vi "Draw Stats.vi"(10 "Stats":T1={"Transform And Project Duration"=0.0, "Raster Duration"=0.0, "Present Duration"=82.5692473, "Frame Rate"=111.70812900055276, "Visible Triangles"=0} {"Frame Rate" format="%.0p"; "Present Duration" format="%.0p"; "Raster Duration" format="%.0p"; "Transform And Project Duration" format="%.0p"}, 11 "Screen in":picture) -> (3 "Screen out":picture)   [LabVIEW 2022 SP3, in "Application.lvlib"]
uses:
  Application.lvlib
  Scene/Stats.ctl
  Libraries/Utility/Utility.lvlib
  Scene/Scene.lvclass
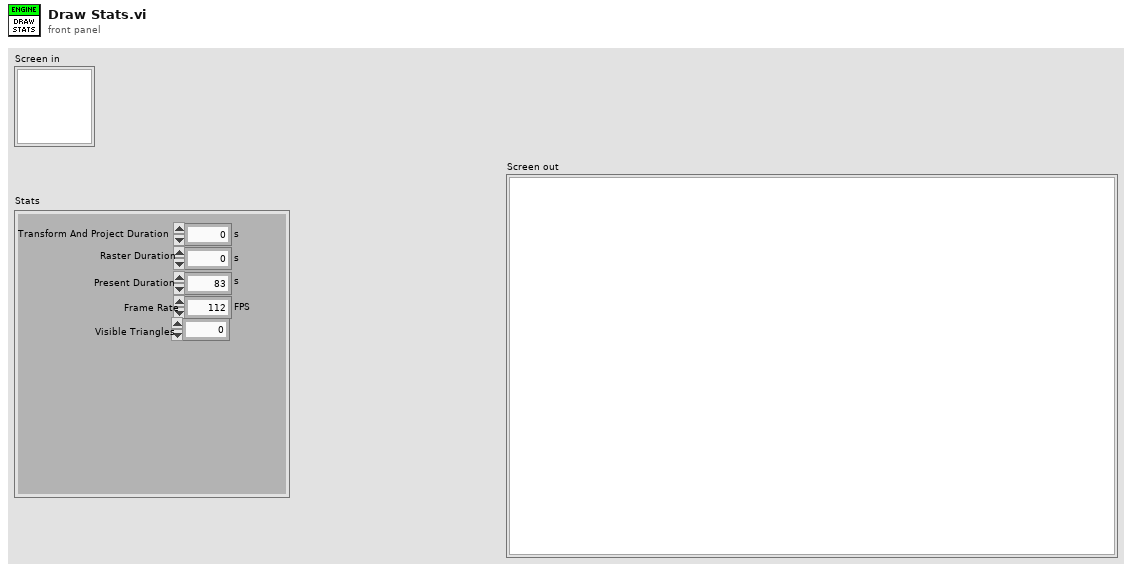
[diagram p1: front panel]
types:
  T1 = typedef "Application.lvlib/Scene.lvclass/Stats.ctl" = cluster{"Transform And Project Duration":dbl, "Raster Duration":dbl, "Present Duration":dbl, "Frame Rate":dbl, "Visible Triangles":i32}
  T2 = cluster{"horizontal":enum16{"left", "center", "right"}, "vertical":enum16{"top", "center", "bottom"}}
  T3 = enum16{"User-specified Font", "Application Font", "System Font", "Dialog Font"}
  T4 = cluster{"Font Name:":string, "Size":i16, "Strikeout?":bool, "Italic?":bool, "Underline?":bool, "Outline?":bool, "Shadow?":bool, "Bold?":bool}
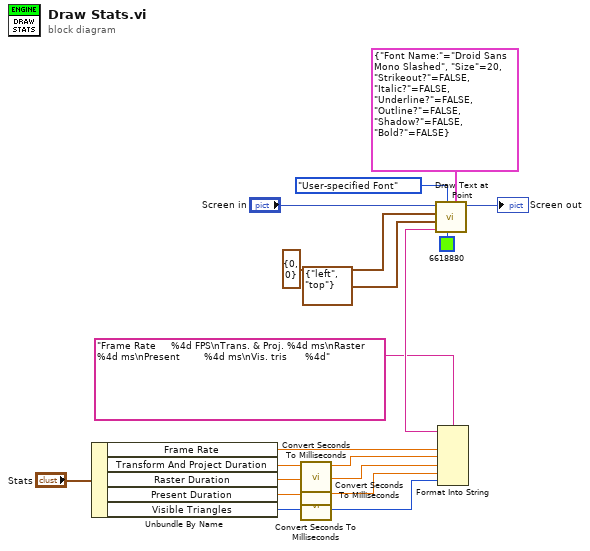
[diagram p0: block diagram]
diagram:
  n1 = Unbundle By Name("Stats") -> ("Frame Rate"=w8:dbl, "Transform And Project Duration"=w6:dbl, "Raster Duration"=w4:dbl, "Present Duration"=w2:dbl, "Visible Triangles"=w7:i32)
  n2 = call "Convert Seconds To Milliseconds.vi"("Seconds"=w6) -> ("Milliseconds"=w5:dbl)  [unwired: 10 in]
  n3 = call "Convert Seconds To Milliseconds.vi"("Seconds"=w4) -> ("Milliseconds"=w3:dbl)  [unwired: 10 in]
  n4 = call "Convert Seconds To Milliseconds.vi"("Seconds"=w2) -> ("Milliseconds"=w1:dbl)  [unwired: 10 in]
  n5 = Format Into String(format string="Frame Rate     %4d FPS\nTrans. & Proj. %4d ms\nRaster         %4d ms\nPresent        %4d ms\nVis. tris      %4d", w8, w5, w3, w1, w7) -> (resulting string=w16:string)  [unwired: 2 in, 1 out]
  n6 = call <vilib>:"Draw Text at Point.vi"("[user-specified font]"=T4 {"Font Name:"="Droid Sans Mono Slashed", "Size"=20, "Strikeout?"=FALSE, "Italic?"=FALSE, "Underline?"=FALSE, "Outline?"=FALSE, "Shadow?"=FALSE, "Bold?"=FALSE}, "text color(black)"=u32 6618880, "desired font(Application)"=T3."User-specified Font", "text"=w16, "alignment(left, top)"=T2 {"horizontal"=enum."left", "vertical"=enum."top"}, "origin"=cluster{"x":i16, "y":i16} {"x"=0, "y"=0}, "picture"="Screen in") -> ("new picture"=→"Screen out":picture)  [unwired: 3 in, 1 out]
